vi "reset_piezo.vi"() -> ()   [LabVIEW 2017]
uses:
  <vilib>/Analysis/Matrix/Datatypes/RealMatrix.ctl
  <vilib>/userdefined/High Color/nirio_resource_hc.ctl
  <vilib>/Analysis/Matrix/Numeric/Conversions/Matrix To Array - RM.vi
  <vilib>/FPGAPlugInAG/cRIO-9082/niLvFpga_Open_cRIO-9082.vi
  <vilib>/rvi/interface/common/dynamic/niFpgaDynamicAddResources.vi
  <vilib>/FPGAPlugInAG/Dynamic/niLvFpga_Reset_Dynamic.vi
  <vilib>/rvi/interface/common/niFpgaWaitOnOcc.vi
  <vilib>/Utility/error.llb/Error Cluster From Error Code.vi
  <vilib>/rvi/errors/niLvFpgaAdjustHostInterfaceError.vi
  <vilib>/FPGAPlugInAG/Dynamic/niLvFpga_Run_Dynamic.vi
  <vilib>/Analysis/Matrix/Numeric/Conversions/Array To Matrix - RA2.vi
  <vilib>/FPGAPlugInAG/Dynamic/niLvFpga_Close_Dynamic.vi
  <vilib>/rvi/interface/nirviOpenFPGA/nirviOpenFPGA.xnode
  FPGA Bitfiles/XYpeizocontrol_FPGATargetSPARTA_nPointidslewOLFI_Q7UGYaeAAEs.lvbitx
  <vilib>/rvi/interface/nirviMethod/nirviMethod.xnode
  <vilib>/rvi/interface/nirviReadWriteControl/nirviReadWriteControl.xnode
  <vilib>/rvi/interface/nirviCloseFPGA/nirviCloseFPGA.xnode
  <vilib>/rvi/errors/niLvFpgaMergeErrorWithErrorCode.vi
  NiFpgaLv.dll
  <vilib>/FPGAPlugInAG/Dynamic/niLvFpga_ConfigureFifo_Dynamic.vi
  <vilib>/rvi/interface/Simulation/niFpgaSimulationCallBeginRW.vi
  <vilib>/FPGAPlugInAG/Dynamic/niLvFpga_WriteFifo_Dynamic.vi
  <vilib>/FPGAPlugInAG/Dynamic/niLvFpga_ReadFifo_Dynamic.vi
  <vilib>/Utility/file.llb/Read Delimited Spreadsheet (DBL).vi
  <vilib>/Analysis/Matrix/NI_Matrix.lvlib
  <vilib>/Utility/file.llb/Write Delimited Spreadsheet (DBL).vi
panel:
  out "stage_data_out":T1
  in  "u_in":T1
  out "Timed Out?":bool
  out "Waveform Graph":dbl[](graph)
  out "Actual Depth 2":u32
  out "unsigned 16bit integer":u16
  out "Elements Remaining":u32
  out "Actual Depth":u32
  out "error out":errorcluster
  out "size(s) 3":i32[](array[numeric])
  out "x+y":i32
  out "YK TO":bool
  out "Unstable Traj":bool
  in  "traj_in_path":path
  out "size(s) 2":i32[](array[numeric])
  in  "data_out_path":path
  out "Loop Done":bool
  in  "Abort":bool
  in  "TsTicks":u32=1600
  out "y iter":i32
  out "size(s)":i32
  in  "umax":dbl=4.0 format="%#_13g"
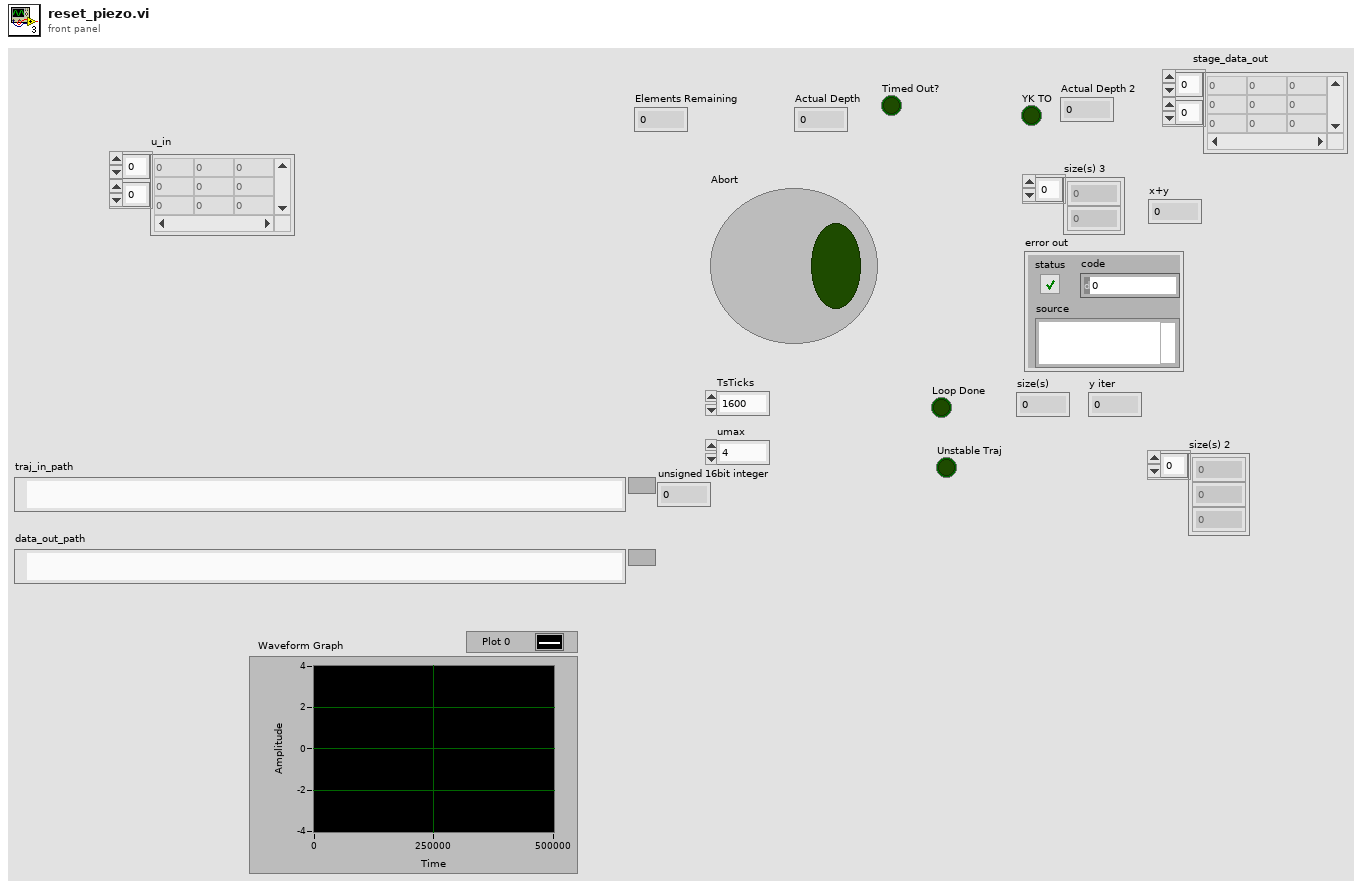
[diagram p1: front panel]
types:
  T1 = typedef "NI_Matrix.lvlib/RealMatrix.ctl" = dbl[][]
  T2 = typedef "nirio_resource_hc.ctl" = tag
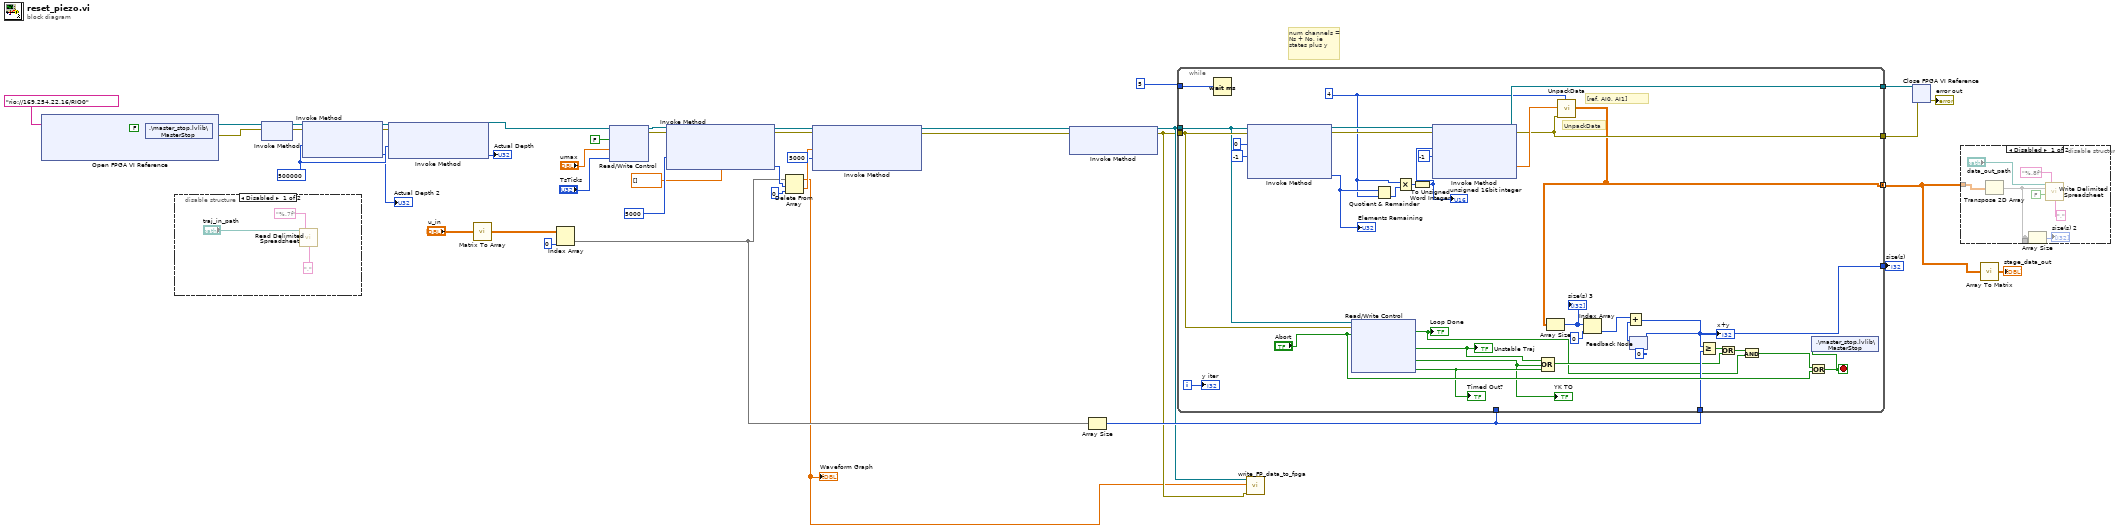
[diagram p0: block diagram]
diagram:
  w31 = 500000
  # "num channels = Ns + No, ie states plus y"
  n1 = xnode "Open FPGA VI Reference"("resource name"=T2 "rio://169.254.22.16/RIO0") -> ("FPGA VI Reference Out"=w39:refnum<k20>, "error out"=w8:errorcluster)  [unwired: 1 in]
  n2 = shared-variable ".\\master_stop.lvlib\\MasterStop"(FALSE ("MasterStop"), error in=w8) -> (error out=w7:errorcluster)
  n3 = disable-structure shown="Disabled" {
    frame Disabled {
      n4 = call-poly <vilib>:"Read Delimited Spreadsheet.vi"("file path (dialog if empty)"="traj_in_path", "format (%.3f)"="%.7f", "delimiter (\\t)"="," ("delimiter (\\t)")) -> ()  [unwired: 7 in, 6 out]
    }
    frame Enabled {
    }
  }
  n5 = xnode "Invoke Method"("FPGA VI Reference In"=w39, "error in"=w7) -> ("FPGA VI Reference Out"=w37:refnum<k20>, "error out"=w36:errorcluster)
  n6 = xnode "Invoke Method"("FPGA VI Reference In"=w37, "error in"=w36, "Requested Depth"=w31) -> ("FPGA VI Reference Out"=w33:refnum<k20>, "error out"=w32:errorcluster, "Actual Depth"=→"Actual Depth 2":u32)
  n7 = xnode "Invoke Method"("FPGA VI Reference In"=w33, "error in"=w32, "Requested Depth"=w31) -> ("FPGA VI Reference Out"=w25:refnum<k20>, "Actual Depth"=→"Actual Depth":u32)  [unwired: 1 out]
  n8 = call-poly <vilib>:"Matrix To Array.vi"("Real Matrix"="u_in") -> ("Real 2D Array"=w3:dbl[][])
  n9 = Index Array(array=w3, index (col)=0 ("disabled index (col)")) -> (element=w12:dbl[])  [unwired: 1 in]
  n10 = xnode "Read/Write Control"("FPGA VI Reference In"=w25, "Abort"=FALSE, "ymax"="umax", "TsTicks"="TsTicks") -> ("FPGA VI Reference Out"=w24:refnum<k20>, "error out"=w23:errorcluster)  [unwired: 1 in]
  n11 = xnode "Invoke Method"("FPGA VI Reference In"=w24, "error in"=w23, "Data"=sgl[] [], "Timeout (ms)"=5000) -> ("FPGA VI Reference Out"=w20:refnum<k20>, "error out"=w19:errorcluster, "Empty Elements Remaining"=w14:u32)
  n12 = Delete From Array(array=w12, length=w14, index=0) -> (deleted portion=w15:dbl[], array with subset deleted=w5:dbl[])
  "Waveform Graph" <- w5
  n13 = xnode "Invoke Method"("FPGA VI Reference In"=w20, "error in"=w19, "Data"=w15, "Timeout (ms)"=5000) -> ("FPGA VI Reference Out"=w18:refnum<k20>, "error out"=w17:errorcluster)  [unwired: 1 out]
  n14 = xnode "Invoke Method"("FPGA VI Reference In"=w18, "error in"=w17) -> ("FPGA VI Reference Out"=w11:refnum<k20>, "error out"=w6:errorcluster)  [unwired: 1 in]
  n15 = Array Size(array=w12) -> (size(s)=w29:i32)
  n16 = while {
    tunnel: 5 -> [w81]
    tunnel: w11 -> [w61]
    tunnel: w6 -> [w62]
    tunnel: [w54] -> w34
    tunnel: [w73] -> w41
    tunnel: [w59] -> w40
    tunnel: [w52] -> w1 mode=concatenating
    tunnel: w29 -> [_]
    tunnel: w29 -> [w58]
    i -> [w64]
    stop <- w53 stop-if-true
    w63 = u32 4 ("y")
    # "[ref, AI0, AI1]"
    # "UnpackData"
    n17 = Wait (ms)(milliseconds to wait=w81) -> ()  [unwired: 1 out]
    n18 = xnode "Invoke Method"("FPGA VI Reference In"=w61, "error in"=w62, "Number of Elements"=0 ("Timeout (ms)"), "Timeout (ms)"=-1) -> ("FPGA VI Reference Out"=w77:refnum<k20>, "error out"=w78:errorcluster, "Elements Remaining"=w70:u32)  [unwired: 1 out]
    "Elements Remaining" <- w70
    n19 = xnode "Read/Write Control"("FPGA VI Reference In"=w61, "error in"=w62, "Abort"="Abort") -> ("Loop Done"=w47:bool, "Unstable Traj"=w48:bool, "YK TO"=w49:bool, "Timed Out?"=w50:bool)  [unwired: 2 out]
    "Loop Done" <- w47
    "Unstable Traj" <- w48
    "YK TO" <- w49
    "Timed Out?" <- w50
    n20 = Quotient & Remainder(x=w70, y=w63) -> (floor(x/y)=w71:u32)  [unwired: 1 out]
    n21 = Multiply(x=w63, y=w71) -> (x*y=w75:u32)
    n22 = To Unsigned Word Integer(number=w75) -> (unsigned 16bit integer=w72:u16)
    "unsigned 16bit integer" <- w72
    n23 = xnode "Invoke Method"("FPGA VI Reference In"=w77, "error in"=w78, "Number of Elements"=w72, "Timeout (ms)"=-1) -> ("FPGA VI Reference Out"=w73:refnum<k20>, "error out"=w54:errorcluster, "Data"=w69:sgl[])  [unwired: 1 out]
    n24 = Compound Arithmetic op=OR(w48, w49, w50) -> (w51:bool)
    n25 = call "UnpackData.vi"("NumChannels"=w63, "error In"=w54, "1D Data In"=w69) -> ("2D Data Out"=w52:dbl[][])  [unwired: 7 in, 1 out]
    n26 = Array Size(array=w52) -> (size(s)=w68:i32[])
    "size(s) 3" <- w68
    n27 = Index Array(array=w68, index=0) -> (element=w66:i32)
    n28 = feedback #1(0) -> (w67:i32)
    n29 = Add(x=w66, y=w67) -> (x+y=w59:i32)
    "x+y" <- w59
    n30 = feedback-in #1(w59) -> ()
    n31 = Greater Or Equal?(x=w59, y=w58) -> (x >= y?=w57:bool)
    n32 = Or(x=w57, y=w51) -> (x .or. y?=w56:bool)
    n33 = And(x=w56, y=w47) -> (x .and. y?=w55:bool)
    n34 = Or(x=w55, y="Abort") -> (x .or. y?=w53:bool)
    n35 = shared-variable ".\\master_stop.lvlib\\MasterStop"(w53) -> ()  [unwired: 1 in, 1 out]
    "y iter" <- w64
  }
  "size(s)" <- w40
  n36 = call "write_FP_data_to_fpga.vi"("error in"=w6, "all rows"=w5, "FPGA Interface"=w11) -> ()  [unwired: 7 in, 2 out]
  n37 = xnode "Close FPGA VI Reference"("FPGA VI Reference In"=w41, "error in"=w34) -> ("error out"=→"error out":errorcluster)
  n38 = disable-structure shown="Disabled" {
    disable-tunnel: w1 -> [w83 _]
    disable-tunnel: [w82 _] -> _
    frame Disabled {
      n39 = Transpose 2D Array(2D array=w83) -> (transposed array=w82:dbl[][])
      n40 = Array Size(array=w82) -> (size(s)=→"size(s) 2":i32[])
      n41 = call-poly <vilib>:"Write Delimited Spreadsheet.vi"("file path (dialog if empty)"="data_out_path", "format (%.3f)"="%.8f", "2D data"=w82, "append to file? (new file:F)"=FALSE, "delimiter (\\t)"="," ("delimiter (\\t)")) -> ()  [unwired: 9 in, 2 out]
    }
    frame Enabled {
    }
  }
  n42 = call-poly <vilib>:"Array To Matrix.vi"("Real 2D Array"=w1) -> ("Real Matrix"=→"stage_data_out":T1)
